vi "SwitchedDMM.vi"(5 "DMM":refnum<class "MIO.lvclass">, 6 "Setting":T1={"Resolution (Digits)"=5.5, "Current Source (Amps)"=0.001, "Range"=2.0, "Measurement Type"=enum."4-wire Resistance"} {"Resolution (Digits)" items=["3 1/2"=3.5, "4 1/2"=4.5, "5 1/2"=5.5, "6 1/2"=6.5, "7 1/2"=7.5]; "Current Source (Amps)" items=["1uA"=1e-06, "10uA"=1e-05, "100uA"=0.0001, "1mA"=0.001]}, 7 "Switch":refnum<class "Switch.lvclass">, 8 "error in":errorcluster, 9 "Connection(s)":string="ch49->com3", 10 "Switch Resource":string, 11 "DMM Resource":string) -> (0 "error out":errorcluster, 1 "Measurements":dbl=7.500284645380634, 2 "DMM out":refnum<class "MIO.lvclass">, 3 "Switch out":refnum<class "Switch.lvclass">)   [LabVIEW 2019, in "Code Modules.lvlib"]
uses:
  PPLs/Hardware Abstraction.lvlibp/Harware Abstraction/Switch/Switch.lvclass
  PPLs/Hardware Abstraction.lvlibp/Harware Abstraction/MultiIO/MIO.lvclass
  Code Modules.lvlib
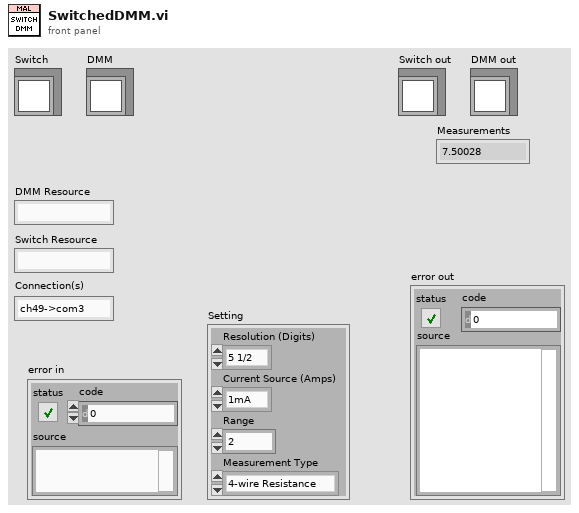
[diagram p1: front panel]
types:
  T1 = cluster{"Resolution (Digits)":dbl, "Current Source (Amps)":dbl, "Range":dbl, "Measurement Type":enum16{"DC Volts", "AC Volts", "DC Current", "AC Current", "2-wire Resistance", "4-wire Resistance", "Diode", "Frequency", "Period", "AC Volts DC Coupled", "Capacitance", "Inductance", "Temperature"}}
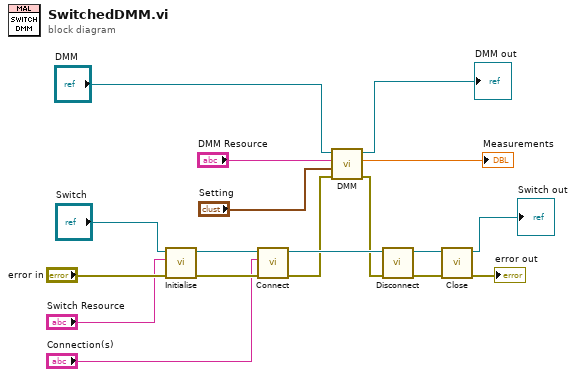
[diagram p0: block diagram]
diagram:
  n1 = call-dynamic "Initialise.vi"("error in (no error)"="error in", "Instrument Ref"="Switch Resource", "Instrument in"="Switch") -> ("error out"=w12:errorcluster, "Instrument out"=w6:refnum<class "Switch.lvclass">)  [unwired: 7 in]
  n2 = call-dynamic "Connect.vi"("error in (no error)"=w12, "Channel(s)"="Connection(s)", "Switch in"=w6) -> ("error out"=w3:errorcluster, "Switch out"=w5:refnum<class "Switch.lvclass">)  [unwired: 7 in]
  n3 = call "DMM.vi"("error in"=w3, "Setting"="Setting", "DMM Ref"="DMM Resource", "DMM"="DMM") -> ("error out"=w2:errorcluster, "Measurements"=→"Measurements":dbl, "DMM"=→"DMM out":refnum<class "MIO.lvclass">)  [unwired: 5 in]
  n4 = call-dynamic "Disconnect.vi"("error in (no error)"=w2, "Switch in"=w5) -> ("error out"=w11:errorcluster, "Switch out"=w4:refnum<class "Switch.lvclass">)  [unwired: 8 in]
  n5 = call-dynamic "Close.vi"("error in (no error)"=w11, "Instrument in"=w4) -> ("error out"=→"error out":errorcluster, "Instrument out"=→"Switch out":refnum<class "Switch.lvclass">)  [unwired: 8 in]
